vi "pointbypoint2vi.vi"() -> ()   [LabVIEW 2016]
uses:
  <vilib>/ptbypt/NI_PtbyPt.lvlib
panel:
  out "appended array":dbl[][](array[numeric])
  out "Waveform Graph":dbl[](graph)
  out "Waveform Chart":dbl(graph)
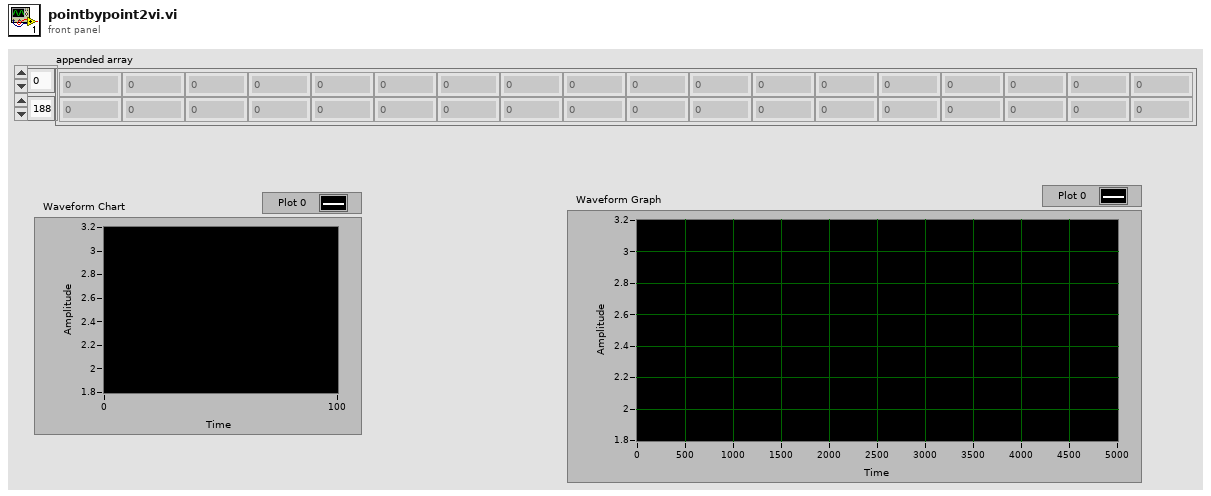
[diagram p1: front panel]
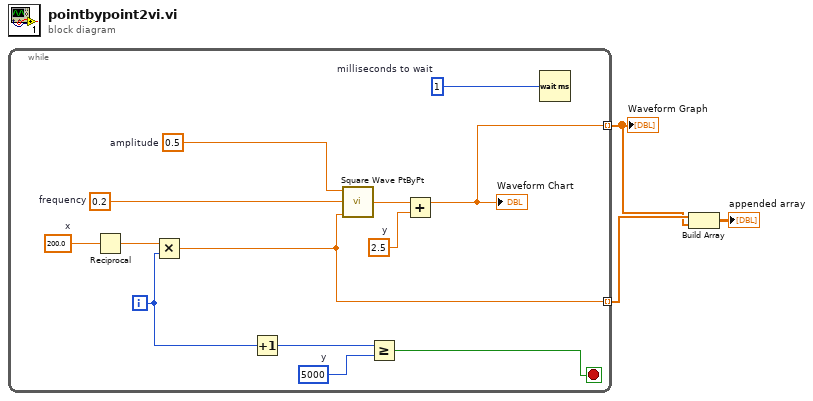
[diagram p0: block diagram]
diagram:
  n1 = while {
    tunnel: [w9] -> w2 mode=indexing
    tunnel: [w11] -> w3 mode=indexing
    i -> [w7]
    stop <- w4 stop-if-true
    w6 = 5000  # y
    w8 = 2.5  # y
    w12 = 200.0  # x
    w15 = u32 1  # milliseconds to wait
    w13 = 0.2  # frequency
    w16 = 0.5  # amplitude
    n2 = Reciprocal(x=w12) -> (1/x=w10:dbl)
    n3 = Multiply(x=w10, y=w7) -> (x*y=w11:dbl)
    n4 = Increment(x=w7) -> (x+1=w5:i32)
    n5 = call <vilib>:"Square Wave PtByPt.vi"("amplitude"=w16, "frequency"=w13, "time"=w11) -> ("square wave"=w14:dbl)  [unwired: 2 in]
    n6 = Greater Or Equal?(x=w5, y=w6) -> (x >= y?=w4:bool)
    n7 = Add(x=w14, y=w8) -> (x+y=w9:dbl)
    "Waveform Chart" <- w9
    n8 = Wait (ms)(milliseconds to wait=w15) -> ()  [unwired: 1 out]
  }
  "Waveform Graph" <- w2
  n9 = Build Array(w3, w2) -> (→"appended array":dbl[][])
